vi "set_item_by_name.vi"(6 "close_item? (true)":bool=TRUE, 8 "error in (no error)":errorcluster, 9 "Item":refnum<class "Item.lvclass">, 10 "item_name":string, 11 "Table in":refnum<class "Table.lvclass">) -> (0 "error out":errorcluster, 3 "Table out":refnum<class "Table.lvclass">)   [LabVIEW 2020, in "toml_edit.lvlib" / "Table.lvclass"]
uses:
  Table.lvclass
  Item/Item.lvclass
  Table.lvclass/Table.ctl
  Item/Item.lvclass/Item.ctl
  dragon_toml_64.dll
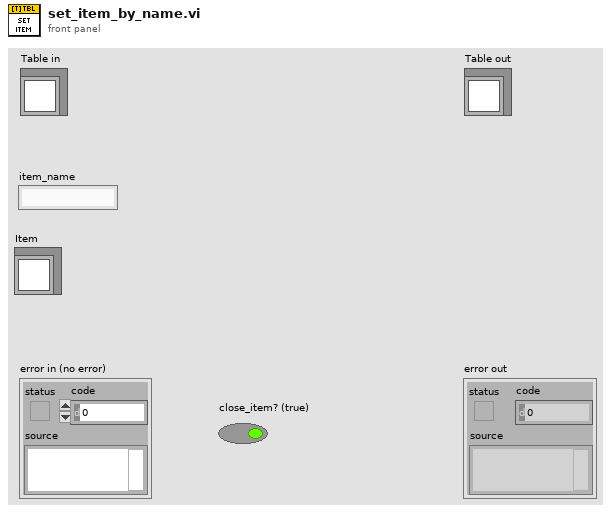
[diagram p1: front panel]
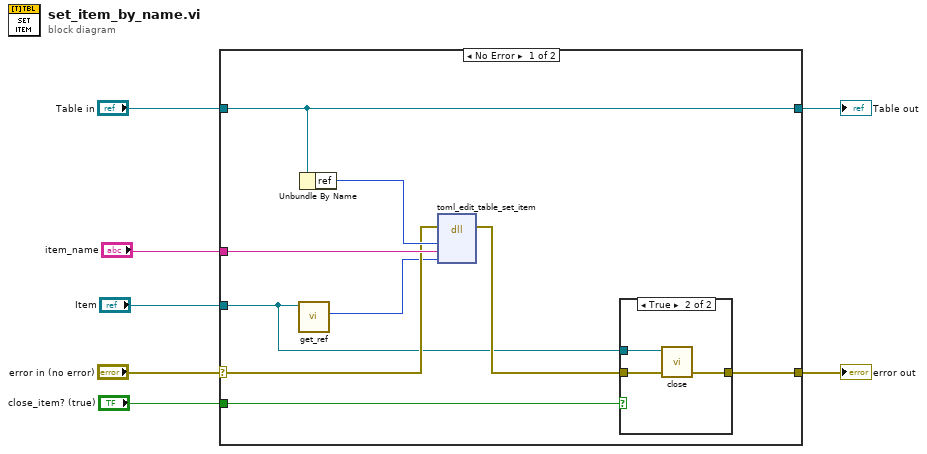
[diagram p0: block diagram]
diagram:
  n1 = case shown="No Error" "error in (no error)" {
    selector: "error in (no error)" -> [w13 w22]
    tunnel: [w10 w22] -> w6
    tunnel: [w16 w21] -> w4
    tunnel: "Table in" -> [w16 w21]
    tunnel: "item_name" -> [w14 _]
    tunnel: "Item" -> [w9 _]
    tunnel: "close_item? (true)" -> [w8 _]
    frame No Error {
      n2 = call "get_ref.vi"("Item in"=w9) -> ("ref"=w12:u64)  [unwired: 10 in]
      n3 = Unbundle By Name(w16) -> ("ref"=w15:u64)
      n4 = dll-call lib="C:/Projects/labview-project-load-tools/source/submodules/toml-edit-labview/lv_src/dragon_toml_*.dll" fn="toml_edit_table_set_item"(error in=w13, "table_ref"=w15, "item_name"=w14, "item_ref"=w12) -> (error out=w11:errorcluster)  [unwired: 6 in, 1 out]
      n5 = case shown="True" w8 {
        tunnel: w11 -> [w17 w20]
        tunnel: [w17 w19] -> w10
        tunnel: w9 -> [_ w18]
        frame False {
        }
        frame True {
          n6 = call "close.vi"("error in (no error)"=w20, "Item in"=w18) -> ("error out"=w19:errorcluster)  [unwired: 9 in]
        }
      }
    }
    frame Error {
    }
  }
  "error out" <- w6
  "Table out" <- w4
